vi "COM String To Real COM.vi"(11 "COM String":string) -> (3 "COM Out":refnum<visa-resource-name>)   [LabVIEW 2021]
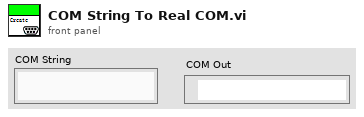
[diagram p1: front panel]
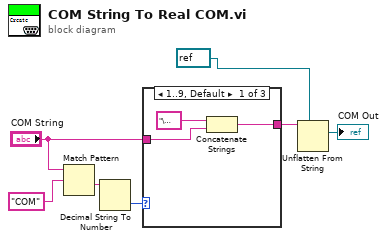
[diagram p0: block diagram]
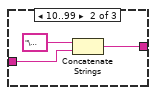
[diagram p2: hidden frame]
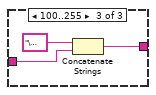
[diagram p3: hidden frame]
diagram:
  n1 = Match Pattern(string="COM String", regular expression="COM") -> (after substring=w6:string)  [unwired: 1 in, 3 out]
  n2 = Decimal String To Number(string=w6) -> (number=w5:i32)  [unwired: 2 in, 1 out]
  n3 = case shown="1..9, Default" w5 {
    tunnel: "COM String" -> [w9 w12 w15]
    tunnel: [w8 w11 w14] -> w3
    frame 1..9, Default {
      n4 = Concatenate Strings("\u0000\u0000\u0000\u0004" ("data string"), w9) -> (w8:string)
    }
    frame 10..99 {
      n5 = Concatenate Strings("\u0000\u0000\u0000\u0005" ("data string"), w12) -> (w11:string)
    }
    frame 100..255 {
      n6 = Concatenate Strings("\u0000\u0000\u0000\u0006" ("data string"), w15) -> (w14:string)
    }
  }
  n7 = Unflatten From String(type=refnum<visa-resource-name> refnum ("COM Port"), binary string=w3) -> (value=→"COM Out":refnum<visa-resource-name>)  [unwired: 3 in, 2 out]
